vi "SAOMM-BinningFixer.vi"(0 "PRAMMS-COMM IN":refnum<visa-resource-name>="Hp\u0000\u0002", 1 "Active Refnum":refnum<vi>, 2 "PrAMS-ACK":refnum<vi>, 5 "Signature":u32, 7 "SendSET":bool=TRUE, 9 "MessageType":cluster{string[], u32[]}={["emtError", "emtAreYouThere", "emtAcknowledgment", "emtGetClientType", "emtClientType", "emtGetImageExposureTime", "emtSetImageExposureTime", "emtImageExposureTime", "emtGetOptimalExposureTime", "emtSetOptimalExposureTime", "emtOptimalExposureTime", "emtGetImageEMGain", "emtSetImageEMGain", "emtImageEMGain", "emtGetFPGACtrl", "emtSetFPGACtrl", "emtFPGACtrl", "emtGetImageWidth", "emtSetImageWidth", "emtImageWidth", "emtGetImageHeight", "emtSetImageHeight", "emtImageHeight", "emtGetImageBinning", "emtSetImageBinning", "emtImageBinning", "emtGetImageDisplayFrameRate", "emtSetImageDisplayFrameRate", "emtImageDisplayFrameRate", "emtGetROIWidth", "emtSetROIWidth", "emtROIWidth", "emtGetROIHeight", "emtSetROIHeight", "emtROIHeight", "emtGetROIXOffset", "emtSetROIXOffset", "emtROIXOffset", "emtGetROIYOffset", "emtSetROIYOffset", "emtROIYOffset", "emtStartAcquisition", "mtStopAcquisition", "emtAcquisitionStarted", "emtAcquisitionStopped", "emtGetFalconImage", "emtFalconImage"], [1, 2, 3, 4, 5, 1001, 1101, 1201, 1002, 1102, 1202, 1003, 1103, 1203, 1004, 1104, 1204, 1005, 1105, 1205, 1006, 1106, 1206, 1007, 1107, 1207, 1008, 1108, 1208, 1009, 1109, 1209, 1010, 1110, 1210, 1011, 1111, 1211, 1012, 1112, 1212, 1130, 1131, 1150, 1151, 1070, 1270]}, 11 "Error IN":errorcluster, 12 "Binning":cluster{"Binning Av":u16, "Binning Ap":u16} {"Binning Ap" items=["1 x 1"=1, "2 x 2"=2, "4 x 4"=4, "5 x 5"=5]; "Binning Av" items=["1 x 1"=1, "2 x 2"=2, "4 x 4"=4, "5 x 5"=5]}, 13 "NAXIS":cluster{"Naxis1":u16, "Naxis2":u16}, 14 "ROI Sizes":T3) -> (4 "PRAMMS-COMM OUT":refnum<visa-resource-name>, 6 "ScaleFactor":dbl format="%.2g", 8 "ROISizesOut":T2, 10 "ROIMinMax":T1, 15 "Error OUT":errorcluster)   [LabVIEW 2019]
uses:
  Polymorphics/Num2littleEndian(U16).vi
panel:
  out "ROIXMax":u16
  out "ROIYMax":u16
  out "ROIXMin":u16
  out "ROIYMin":u16
  out "ROIXOffset OUT":u16
  out "ROIYOffset OUT":u16
  out "ROIWidth OUT":u16
  out "ROIHeight OUT":u16
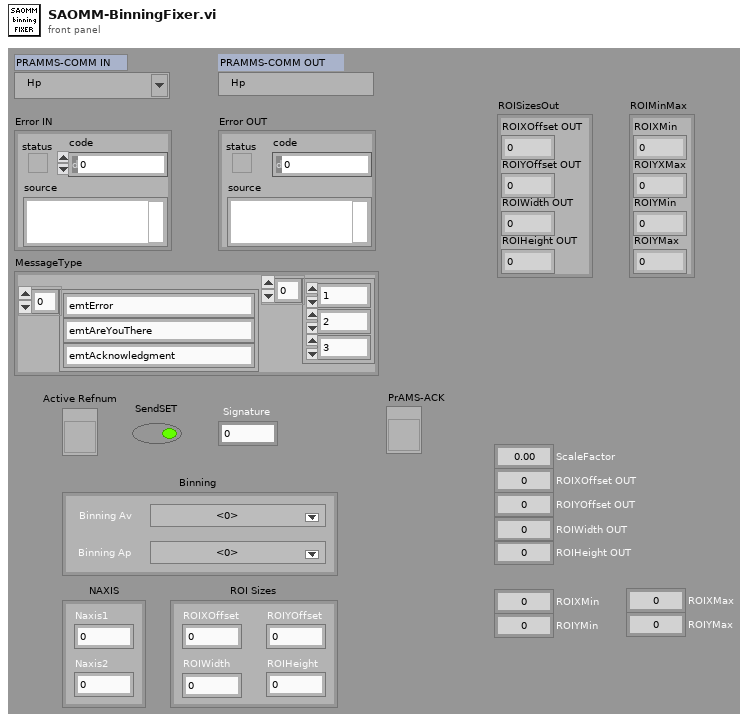
[diagram p1: front panel]
types:
  T1 = cluster{"ROIXMin":u16, "ROIYXMax":u16, "ROIYMin":u16, "ROIYMax":u16}
  T2 = cluster{"ROIXOffset OUT":u16, "ROIYOffset OUT":u16, "ROIWidth OUT":u16, "ROIHeight OUT":u16}
  T3 = cluster{"ROIXOffset":u16, "ROIYOffset":u16, "ROIWidth":u16, "ROIHeight":u16}
  T4 = cluster{"ROIXMin":u16, "ROIXMax":u16, "ROIYMin":u16, "ROIYMax":u16}
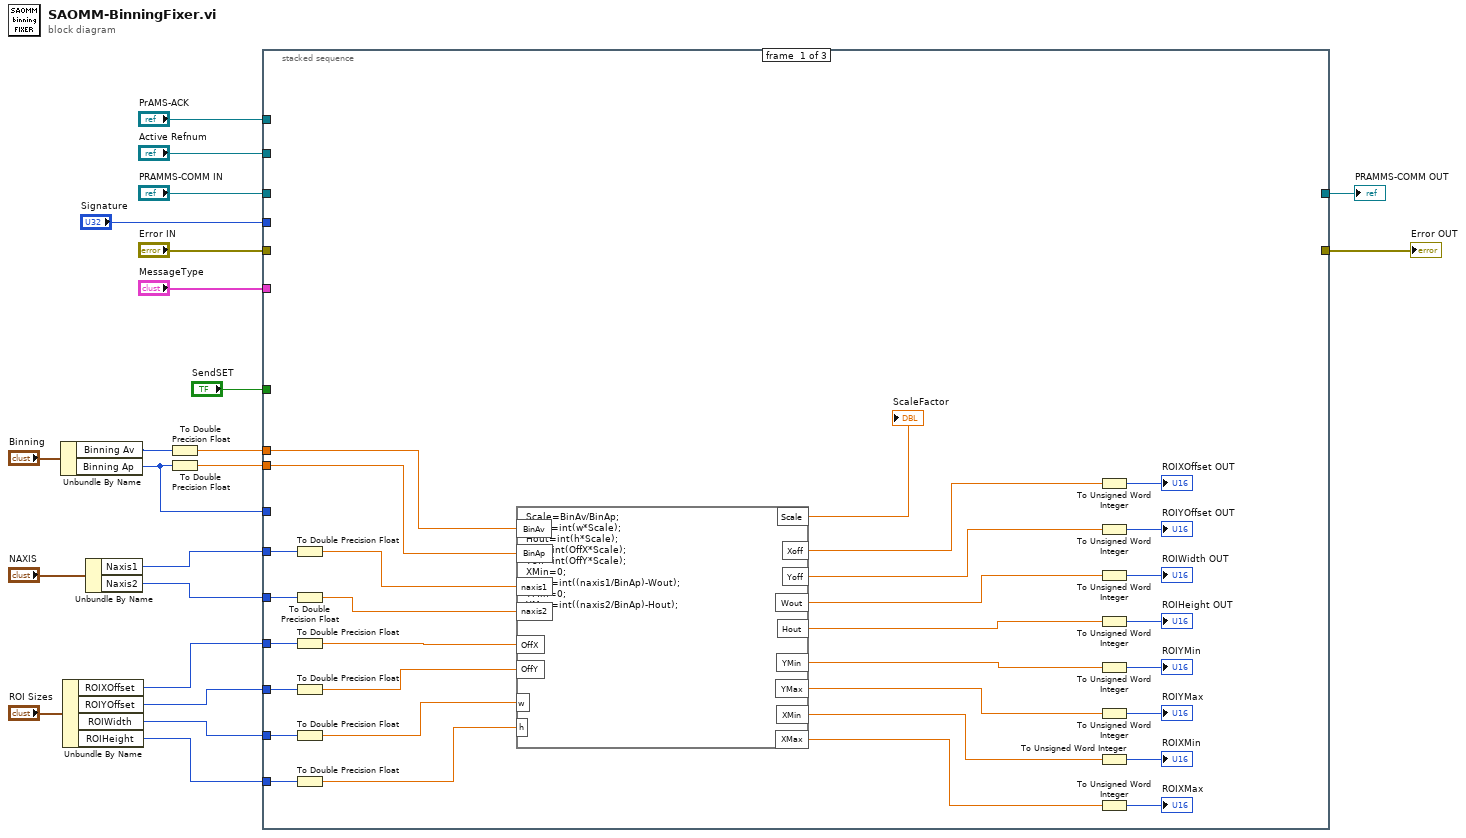
[diagram p0: block diagram]
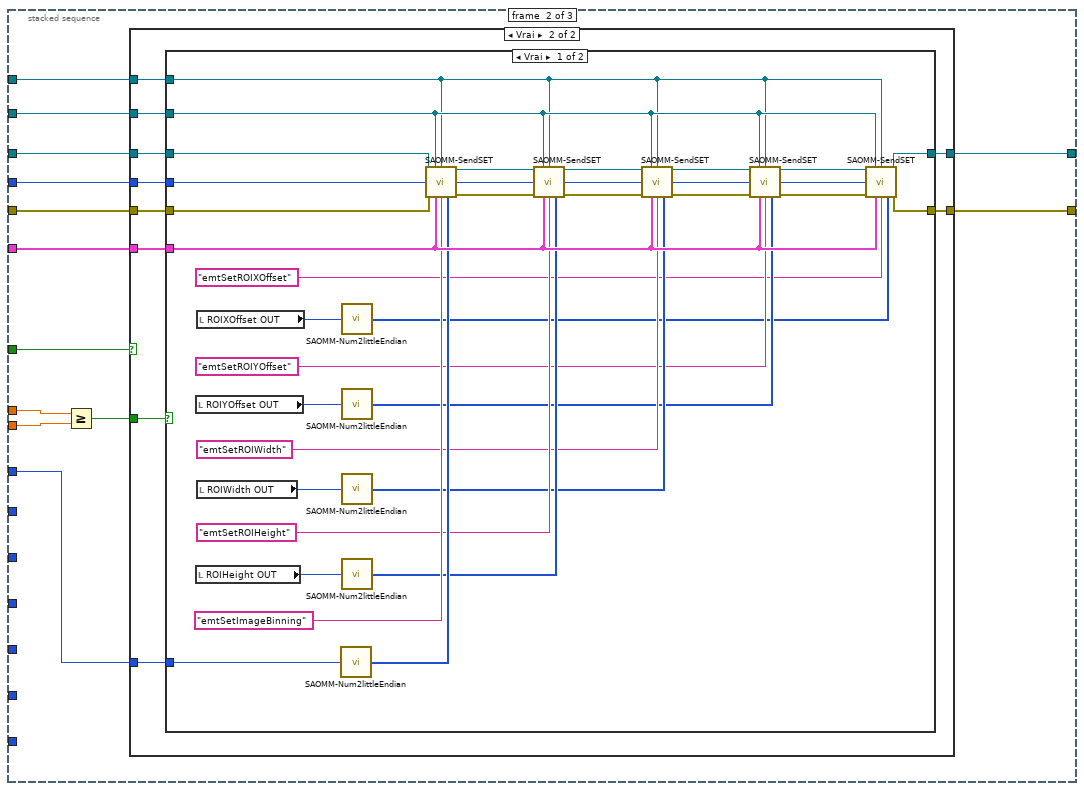
[diagram p2: hidden frame]
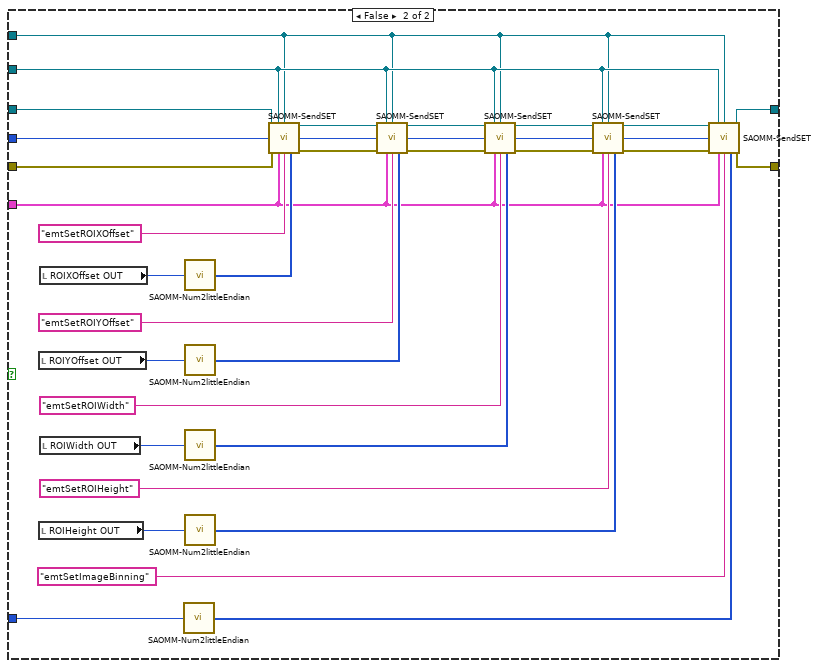
[diagram p4: hidden frame]
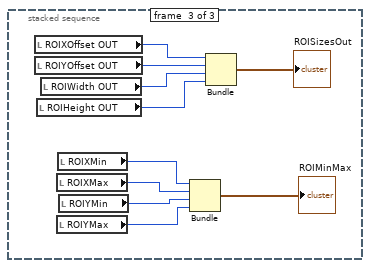
[diagram p5: hidden frame]
diagram:
  n1 = Unbundle By Name("Binning") -> ("Binning Av"=w21:u16, "Binning Ap"=w11:u16)
  n2 = Unbundle By Name("ROI Sizes") -> ("ROIXOffset"=w5:u16, "ROIYOffset"=w4:u16, "ROIWidth"=w3:u16, "ROIHeight"=w2:u16)
  n3 = Unbundle By Name("NAXIS") -> ("Naxis1"=w8:u16, "Naxis2"=w7:u16)
  n4 = To Double Precision Float(number=w21) -> (double precision float=w14:dbl)
  n5 = To Double Precision Float(number=w11) -> (double precision float=w13:dbl)
  n6 = stacked-sequence {
    tunnel: w5 -> [w53 _ _]
    tunnel: w4 -> [w52 _ _]
    tunnel: w3 -> [w51 _ _]
    tunnel: w2 -> [w50 _ _]
    tunnel: w7 -> [w45 _ _]
    tunnel: w8 -> [w44 _ _]
    tunnel: "SendSET" -> [_ w66 _]
    tunnel: "PRAMMS-COMM IN" -> [_ w65 _]
    tunnel: "Error IN" -> [_ w64 _]
    tunnel: "MessageType" -> [_ w63 _]
    tunnel: [_ w60 _] -> w16
    tunnel: [_ w59 _] -> w15
    tunnel: w14 -> [w42 w57 _]
    tunnel: w13 -> [w41 w56 _]
    tunnel: "PrAMS-ACK" -> [_ w62 _]
    tunnel: "Active Refnum" -> [_ w61 _]
    tunnel: w11 -> [_ w54 _]
    tunnel: "Signature" -> [_ w58 _]
    frame #0 {
      n7 = To Double Precision Float(number=w44) -> (double precision float=w40:dbl)
      n8 = To Double Precision Float(number=w45) -> (double precision float=w39:dbl)
      n9 = To Double Precision Float(number=w53) -> (double precision float=w38:dbl)
      n10 = To Double Precision Float(number=w52) -> (double precision float=w37:dbl)
      n11 = To Double Precision Float(number=w51) -> (double precision float=w36:dbl)
      n12 = To Double Precision Float(number=w50) -> (double precision float=w35:dbl)
      n13 = formula code="Scale=BinAv/BinAp;\nWout=int(w*Scale);\nHout=int(h*Scale);\nXoff=int(OffX*Scale);\nYoff=int(OffY*Scale);\nXMin=0;\nXMax=int((naxis1/BinAp)-Wout);\nYMin=0;\nYMax=int((naxis2/BinAp)-Hout);"("BinAv"=w42, "BinAp"=w41, "OffX"=w38, "OffY"=w37, "w"=w36, "h"=w35, "naxis1"=w40, "naxis2"=w39) -> ("Xoff"=w24:dbl, "Yoff"=w34:dbl, "YMin"=w28:dbl, "YMax"=w25:dbl, "XMax"=w23:dbl, "XMin"=w31:dbl, "Scale"=→"ScaleFactor":dbl, "Wout"=w33:dbl, "Hout"=w32:dbl)
      n14 = To Unsigned Word Integer(number=w24) -> (unsigned 16bit integer=→"ROIXOffset OUT":u16)
      n15 = To Unsigned Word Integer(number=w34) -> (unsigned 16bit integer=→"ROIYOffset OUT":u16)
      n16 = To Unsigned Word Integer(number=w33) -> (unsigned 16bit integer=→"ROIWidth OUT":u16)
      n17 = To Unsigned Word Integer(number=w32) -> (unsigned 16bit integer=→"ROIHeight OUT":u16)
      n18 = To Unsigned Word Integer(number=w28) -> (unsigned 16bit integer=→"ROIYMin":u16)
      n19 = To Unsigned Word Integer(number=w25) -> (unsigned 16bit integer=→"ROIYMax":u16)
      n20 = To Unsigned Word Integer(number=w31) -> (unsigned 16bit integer=→"ROIXMin":u16)
      n21 = To Unsigned Word Integer(number=w23) -> (unsigned 16bit integer=→"ROIXMax":u16)
    }
    frame #1 {
      n22 = Greater Or Equal?(x=w57, y=w56) -> (x >= y?=w55:bool)
      n23 = case shown="Vrai" w66 {
        tunnel: w65 -> [w68 w78]
        tunnel: w64 -> [w67 w77]
        tunnel: w63 -> [_ w71]
        tunnel: w61 -> [_ w74]
        tunnel: w62 -> [_ w73]
        tunnel: [w68 w76] -> w60
        tunnel: [w67 w75] -> w59
        tunnel: w58 -> [_ w72]
        tunnel: w55 -> [_ w70]
        tunnel: w54 -> [_ w69]
        frame False {
        }
        frame True {
          n24 = case shown="Vrai" w70 {
            tunnel: w78 -> [w109 w140]
            tunnel: w77 -> [w108 w139]
            tunnel: [w95 w118] -> w76
            tunnel: [w94 w117] -> w75
            tunnel: w74 -> [w93 w116]
            tunnel: w73 -> [w92 w115]
            tunnel: w72 -> [w91 w114]
            tunnel: w71 -> [w90 w113]
            tunnel: w69 -> [w79 w110]
            frame True {
              n25 = local read "ROIYOffset OUT"() -> (w98:u16)
              n26 = local read "ROIHeight OUT"() -> (w100:u16)
              n27 = local read "ROIXOffset OUT"() -> (w101:u16)
              n28 = local read "ROIWidth OUT"() -> (w99:u16)
              n29 = call-poly "SAOMM-Num2littleEndian.vi"("Number"=w79) -> ("LiitleEndianedData"=w89:u8[])  [unwired: 14 in]
              n30 = call-poly "SAOMM-Num2littleEndian.vi"("Number"=w101) -> ("LiitleEndianedData"=w81:u8[])  [unwired: 14 in]
              n31 = call-poly "SAOMM-Num2littleEndian.vi"("Number"=w98) -> ("LiitleEndianedData"=w83:u8[])  [unwired: 14 in]
              n32 = call-poly "SAOMM-Num2littleEndian.vi"("Number"=w99) -> ("LiitleEndianedData"=w85:u8[])  [unwired: 14 in]
              n33 = call-poly "SAOMM-Num2littleEndian.vi"("Number"=w100) -> ("LiitleEndianedData"=w87:u8[])  [unwired: 14 in]
              n34 = call "SAOMM-SendSET.vi"("PRAMMS-COMM IN"=w109, "Active Refnum"=w93, "PrAMS-ACK"=w92, "Signature"=w91, "Error IN"=w108, "MessageType"=w90, "Active SET"="emtSetImageBinning", "Value (little endianed byte array)"=w89) -> ("PRAMMS-COMM OUT"=w107:refnum<visa-resource-name>, "Error OUT"=w106:errorcluster)  [unwired: 4 in, 2 out]
              n35 = call "SAOMM-SendSET.vi"("PRAMMS-COMM IN"=w107, "Active Refnum"=w93, "PrAMS-ACK"=w92, "Signature"=w91, "Error IN"=w106, "MessageType"=w90, "Active SET"="emtSetROIHeight", "Value (little endianed byte array)"=w87) -> ("PRAMMS-COMM OUT"=w105:refnum<visa-resource-name>, "Error OUT"=w104:errorcluster)  [unwired: 4 in, 2 out]
              n36 = call "SAOMM-SendSET.vi"("PRAMMS-COMM IN"=w105, "Active Refnum"=w93, "PrAMS-ACK"=w92, "Signature"=w91, "Error IN"=w104, "MessageType"=w90, "Active SET"="emtSetROIWidth", "Value (little endianed byte array)"=w85) -> ("PRAMMS-COMM OUT"=w103:refnum<visa-resource-name>, "Error OUT"=w102:errorcluster)  [unwired: 4 in, 2 out]
              n37 = call "SAOMM-SendSET.vi"("PRAMMS-COMM IN"=w103, "Active Refnum"=w93, "PrAMS-ACK"=w92, "Signature"=w91, "Error IN"=w102, "MessageType"=w90, "Active SET"="emtSetROIYOffset", "Value (little endianed byte array)"=w83) -> ("PRAMMS-COMM OUT"=w97:refnum<visa-resource-name>, "Error OUT"=w96:errorcluster)  [unwired: 4 in, 2 out]
              n38 = call "SAOMM-SendSET.vi"("PRAMMS-COMM IN"=w97, "Active Refnum"=w93, "PrAMS-ACK"=w92, "Signature"=w91, "Error IN"=w96, "MessageType"=w90, "Active SET"="emtSetROIXOffset", "Value (little endianed byte array)"=w81) -> ("PRAMMS-COMM OUT"=w95:refnum<visa-resource-name>, "Error OUT"=w94:errorcluster)  [unwired: 4 in, 2 out]
            }
            frame False {
              n39 = local read "ROIYOffset OUT"() -> (w129:u16)
              n40 = local read "ROIHeight OUT"() -> (w131:u16)
              n41 = local read "ROIXOffset OUT"() -> (w132:u16)
              n42 = local read "ROIWidth OUT"() -> (w130:u16)
              n43 = call-poly "SAOMM-Num2littleEndian.vi"("Number"=w110) -> ("LiitleEndianedData"=w112:u8[])  [unwired: 14 in]
              n44 = call-poly "SAOMM-Num2littleEndian.vi"("Number"=w132) -> ("LiitleEndianedData"=w128:u8[])  [unwired: 14 in]
              n45 = call-poly "SAOMM-Num2littleEndian.vi"("Number"=w129) -> ("LiitleEndianedData"=w127:u8[])  [unwired: 14 in]
              n46 = call-poly "SAOMM-Num2littleEndian.vi"("Number"=w130) -> ("LiitleEndianedData"=w126:u8[])  [unwired: 14 in]
              n47 = call-poly "SAOMM-Num2littleEndian.vi"("Number"=w131) -> ("LiitleEndianedData"=w125:u8[])  [unwired: 14 in]
              n48 = call "SAOMM-SendSET.vi"("PRAMMS-COMM IN"=w140, "Active Refnum"=w116, "PrAMS-ACK"=w115, "Signature"=w114, "Error IN"=w139, "MessageType"=w113, "Active SET"="emtSetROIXOffset", "Value (little endianed byte array)"=w128) -> ("PRAMMS-COMM OUT"=w138:refnum<visa-resource-name>, "Error OUT"=w137:errorcluster)  [unwired: 4 in, 2 out]
              n49 = call "SAOMM-SendSET.vi"("PRAMMS-COMM IN"=w138, "Active Refnum"=w116, "PrAMS-ACK"=w115, "Signature"=w114, "Error IN"=w137, "MessageType"=w113, "Active SET"="emtSetROIYOffset", "Value (little endianed byte array)"=w127) -> ("PRAMMS-COMM OUT"=w136:refnum<visa-resource-name>, "Error OUT"=w135:errorcluster)  [unwired: 4 in, 2 out]
              n50 = call "SAOMM-SendSET.vi"("PRAMMS-COMM IN"=w136, "Active Refnum"=w116, "PrAMS-ACK"=w115, "Signature"=w114, "Error IN"=w135, "MessageType"=w113, "Active SET"="emtSetROIWidth", "Value (little endianed byte array)"=w126) -> ("PRAMMS-COMM OUT"=w134:refnum<visa-resource-name>, "Error OUT"=w133:errorcluster)  [unwired: 4 in, 2 out]
              n51 = call "SAOMM-SendSET.vi"("PRAMMS-COMM IN"=w134, "Active Refnum"=w116, "PrAMS-ACK"=w115, "Signature"=w114, "Error IN"=w133, "MessageType"=w113, "Active SET"="emtSetROIHeight", "Value (little endianed byte array)"=w125) -> ("PRAMMS-COMM OUT"=w120:refnum<visa-resource-name>, "Error OUT"=w119:errorcluster)  [unwired: 4 in, 2 out]
              n52 = call "SAOMM-SendSET.vi"("PRAMMS-COMM IN"=w120, "Active Refnum"=w116, "PrAMS-ACK"=w115, "Signature"=w114, "Error IN"=w119, "MessageType"=w113, "Active SET"="emtSetImageBinning", "Value (little endianed byte array)"=w112) -> ("PRAMMS-COMM OUT"=w118:refnum<visa-resource-name>, "Error OUT"=w117:errorcluster)  [unwired: 4 in, 2 out]
            }
          }
        }
      }
    }
    frame #2 {
      n53 = local read "ROIXOffset OUT"() -> (w147:u16)
      n54 = local read "ROIYOffset OUT"() -> (w148:u16)
      n55 = local read "ROIHeight OUT"() -> (w150:u16)
      n56 = local read "ROIWidth OUT"() -> (w149:u16)
      n57 = local read "ROIXMax"() -> (w144:u16)
      n58 = local read "ROIYMax"() -> (w142:u16)
      n59 = local read "ROIXMin"() -> (w145:u16)
      n60 = local read "ROIYMin"() -> (w143:u16)
      n61 = Bundle("ROIXMin"=w145, "ROIXMax"=w144, "ROIYMin"=w143, "ROIYMax"=w142) -> (→"ROIMinMax":T4)  [unwired: 1 in]
      n62 = Bundle("ROIXOffset OUT"=w147, "ROIYOffset OUT"=w148, "ROIWidth OUT"=w149, "ROIHeight OUT"=w150) -> (→"ROISizesOut":T2)  [unwired: 1 in]
    }
  }
  "Error OUT" <- w15
  "PRAMMS-COMM OUT" <- w16
